vi "UpdateRefs.vi"(8 "Error In":errorcluster, 10 "VI Ref In":refnum<vi>, 11 "UI Refs in":T1) -> (0 "Error Out":errorcluster, 3 "UI Refs out":T1)   [LabVIEW 2015]
uses:
  Controls & Type Defs/UI Data.ctl
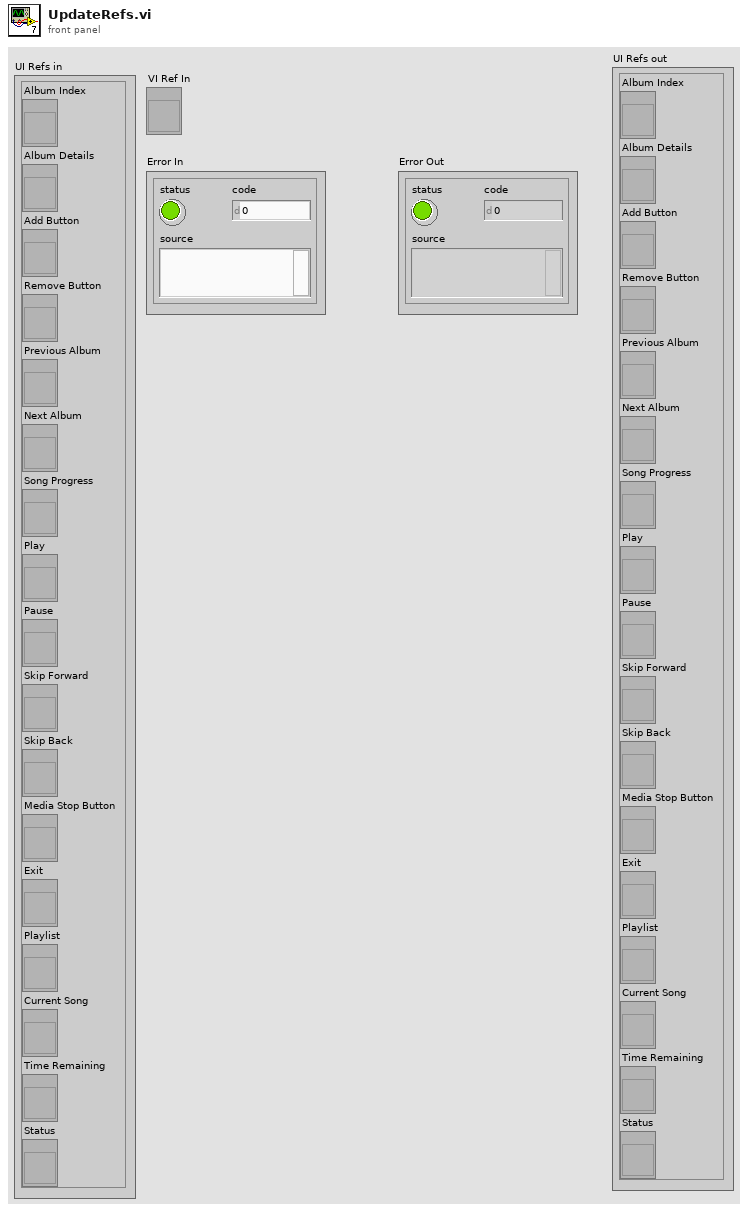
[diagram p1: front panel]
types:
  T1 = typedef "UI Data.ctl" = cluster{"Album Index":refnum<vi>, "Album Details":refnum<vi>, "Add Button":refnum<vi>, "Remove Button":refnum<vi>, "Previous Album":refnum<vi>, "Next Album":refnum<vi>, "Song Progress":refnum<vi>, "Play":refnum<vi>, "Pause ":refnum<vi>, "Skip Forward":refnum<vi>, "Skip Back":refnum<vi>, "Media Stop Button":refnum<vi>, "Exit":refnum<vi>, "Playlist":refnum<vi>, "Current Song":refnum<vi>, "Time Remaining":refnum<vi>, "Status":refnum<vi>}
  T2 = cluster{"[0]":refnum<vi>, "[1]":refnum<vi>, "[2]":refnum<vi>, "[3]":refnum<vi>, "[4]":refnum<vi>, "[5]":refnum<vi>, "[6]":refnum<vi>, "[7]":refnum<vi>, "[8]":refnum<vi>, "[9]":refnum<vi>, "[10]":refnum<vi>, "[11]":refnum<vi>, "[12]":refnum<vi>, "[13]":refnum<vi>, "[14]":refnum<vi>, "[15]":refnum<vi>, "[16]":refnum<vi>}
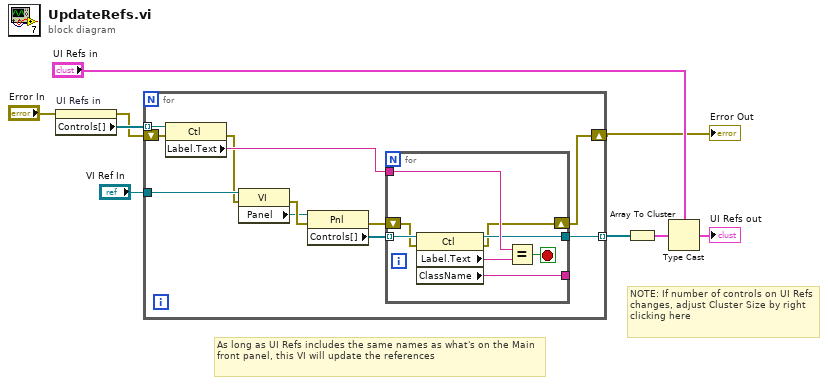
[diagram p0: block diagram]
diagram:
  # "NOTE: If number of controls on UI Refs changes, adjust Cluster Size by right clicking here"
  # "As long as UI Refs includes the same names as what's on the Main front panel, this VI will update the references"
  n1 = property on="UI Refs in" class="Clust (strict)"(error in="Error In") -> (error out=w2:errorcluster, "Controls[]"=w3:refnum<vi>[])  [unwired: 1 in, 1 out]
  n2 = for {
    tunnel: "VI Ref In" -> [w20]
    tunnel: w3 -> [w14] mode=indexing
    tunnel: [w12] -> w8 mode=indexing
    shift-right: [w11] -> w4
    shift-left: w2 -> [w10]
    n3 = property class="Ctl"(reference=w14, error in=w10) -> (error out=w15:errorcluster, "Label.Text"=w18:string)  [unwired: 1 out]
    n4 = property class="VI"(reference=w20, error in=w15) -> (error out=w16:errorcluster, "Panel"=w13:refnum<vi>)  [unwired: 1 out]
    n5 = property class="Pnl"(reference=w13, error in=w16) -> (error out=w17:errorcluster, "Controls[]"=w19:refnum<vi>[])  [unwired: 1 out]
    n6 = for {
      tunnel: w19 -> [w28] mode=indexing
      tunnel: w18 -> [w25]
      shift-right: [w22] -> w11
      shift-left: w17 -> [w26]
      tunnel: [w24] -> w12
      tunnel: [w21] -> _
      stop <- w23 stop-if-true
      n7 = property class="Ctl"(reference=w28, error in=w26) -> (reference out=w24:refnum<vi>, error out=w22:errorcluster, "Label.Text"=w27:string, "ClassName"=w21:string)
      n8 = Equal?(x=w25, y=w27) -> (x = y?=w23:bool)
    }
  }
  "Error Out" <- w4
  n9 = Array To Cluster(array=w8) -> (cluster=w6:T2)
  n10 = Type Cast(type="UI Refs in", x=w6) -> (*(type *) &x=→"UI Refs out":T1)
